vi "Weird Slave.vi"() -> ()   [LabVIEW 2012]
uses:
  API/Slave/Modbus Slave.lvclass
  Data Model/Standard Data Model/Standard Data Model.lvclass
  Transmission Data Unit/RTU/RTU Data Unit.lvclass
  Transmission Data Unit/ASCII/ASCII Data Unit.lvclass
  Network Protocol/Network Slave/TCP/TCP Slave.lvclass
  Transmission Data Unit/Serial Interface/Serial Data Unit.lvclass
  Data Model/Identification Parameters.ctl
  Data Model/Device Data Model.lvclass
  Master Function Definition/Read Device ID code.ctl
panel:
  in  "Port":u16=502
  in  "Serial Type":enum16{"RTU", "ASCII"}(ring)
  in  "Unit ID":u8=1
  in  "HR to write":u16[](array[numeric])=[1, 65535, 40000, 20000]
  in  "Set HR":bool
  in  "Set IR":bool
  in  "IR to write":u16[](array[numeric])=[1, 65535, 40000, 20000]
  in  "IR 6":u16
  in  "Set !":bool
  in  "! status":u8=1
  in  "Set Coils":bool
  in  "Set DI":bool
  in  "DI to write":bool[](array[boolean])=[FALSE, TRUE, FALSE, TRUE]
  in  "coils to write":bool[](array[boolean])=[FALSE, TRUE, FALSE, TRUE]
  in  "set objects":bool
  in  "Objects In":T1[](array[typedef])=[{"Object ID"=0, "Value"="National instruments"}, {"Object ID"=1, "Value"="42"}, {"Object ID"=2, "Value"="1.0.0"}] {"Object ID" format="%x"}
  in  "Coil 6":bool
  out "exception status":u8=1
  out "register values":u16[](array[numeric])=[1, 1, 65535, 40000, 20000, 6]
  out "discrete inputs":bool[](array[boolean])=[FALSE, FALSE, TRUE, FALSE, TRUE, TRUE]
  in  "Read Device ID code":T2
  out "Objects":T1[](array[typedef])=[{"Object ID"=0, "Value"="National instruments"}, {"Object ID"=1, "Value"="42"}, {"Object ID"=2, "Value"="1.0.0"}] {"Object ID" format="%x"}
  in  "Object Id":u8 format="%02x"
  out "holding reg":u16[](array[numeric])=[1, 1, 65535, 40000, 20000, 6]
  out "error out":errorcluster
  in  "stop":bool
  out "Coils":bool[](array[boolean])=[FALSE, FALSE, TRUE, FALSE, TRUE, TRUE] caption="Coils (Master can write coils)"
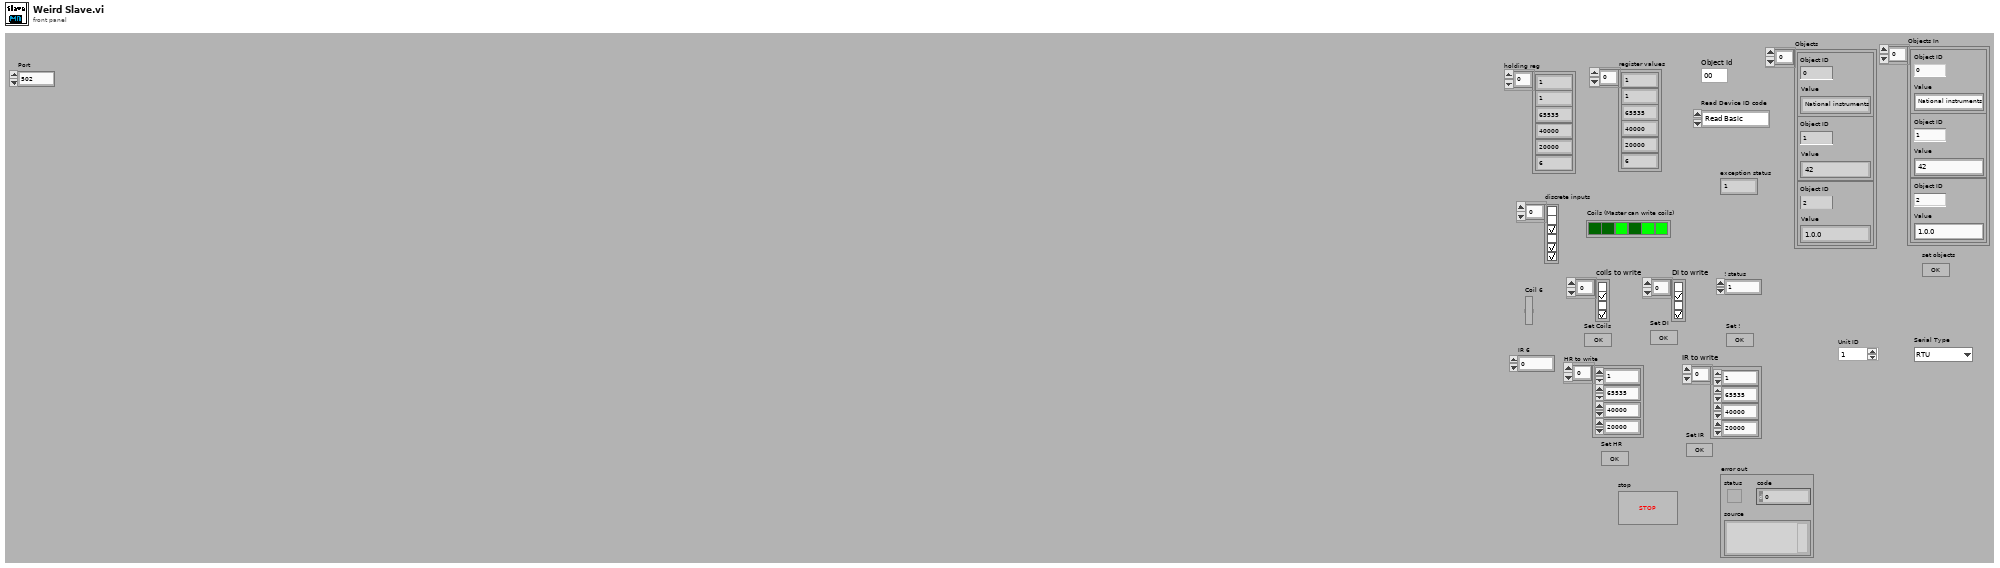
[diagram p1: front panel]
types:
  T1 = typedef "Device Data Model.lvclass/Identification Parameters.ctl" = cluster{"Object ID":u8, "Value":string}
  T2 = typedef "Device Data Model.lvclass/Read Device ID code.ctl" = enum8{"Read Basic", "Read Regular", "Read Extended", "Read Specific"}
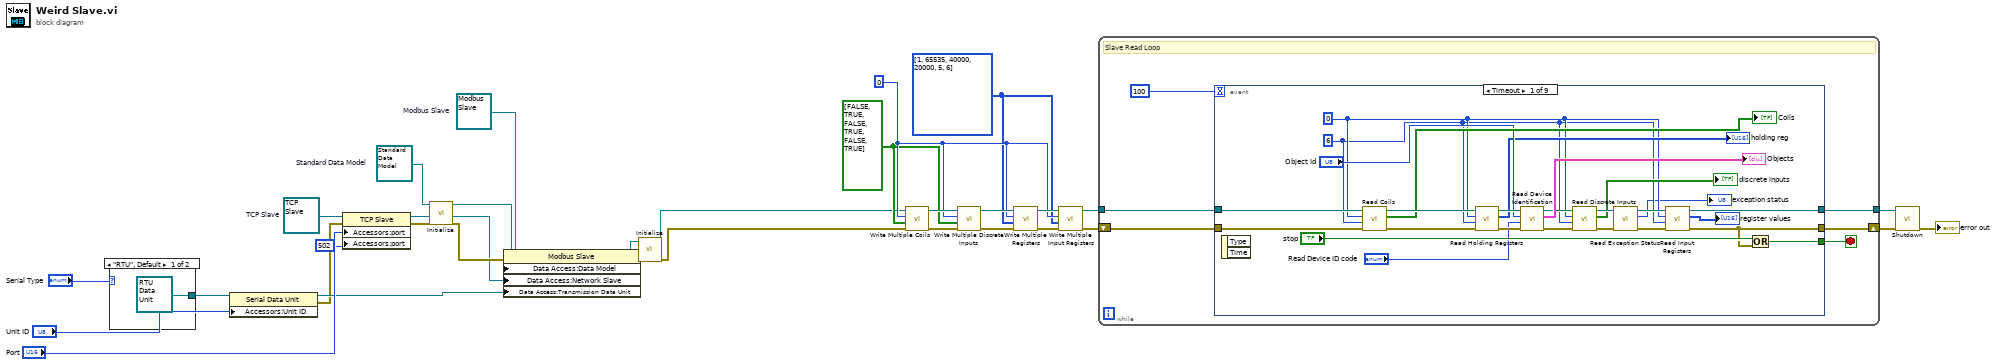
[diagram p0: block diagram]
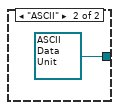
[diagram p2: hidden frame]
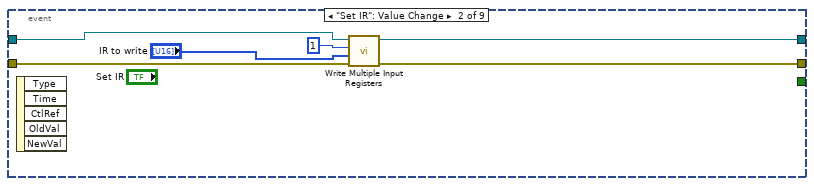
[diagram p3: hidden frame]
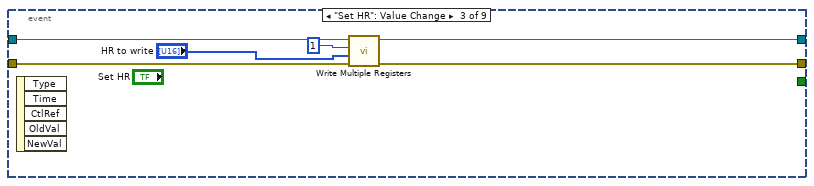
[diagram p4: hidden frame]
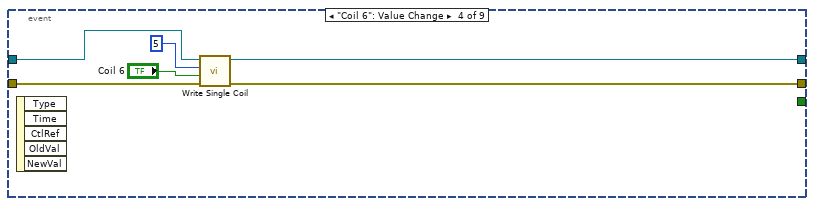
[diagram p5: hidden frame]
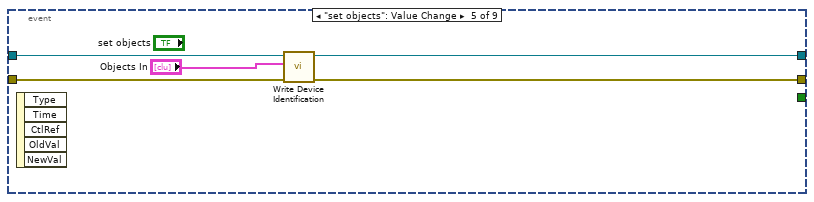
[diagram p6: hidden frame]
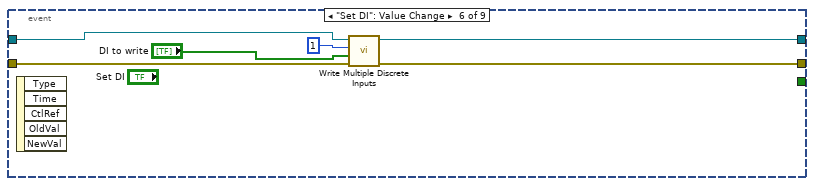
[diagram p7: hidden frame]
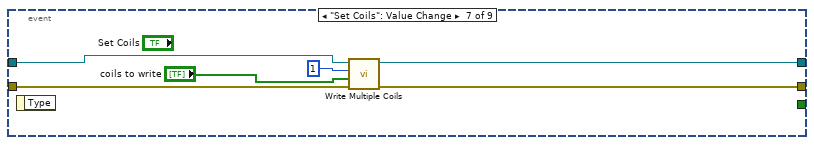
[diagram p8: hidden frame]
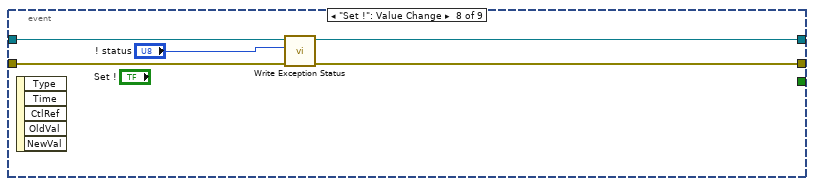
[diagram p9: hidden frame]
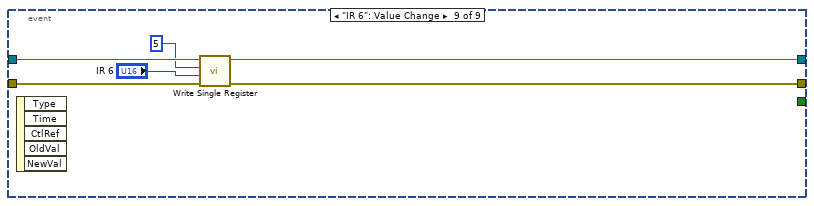
[diagram p10: hidden frame]
diagram:
  w4 = refnum<class "Standard Data Model.lvclass"> refnum  # Standard Data Model
  w15 = refnum<class "TCP Slave.lvclass"> refnum  # TCP Slave
  w13 = refnum<class "Modbus Slave.lvclass"> refnum  # Modbus Slave
  w19 = bool[] [FALSE, TRUE, FALSE, TRUE, FALSE, TRUE] ("coils to write")
  w20 = u16[] [1, 65535, 40000, 20000, 5, 6] ("registers")
  w21 = u16 0 ("starting address")
  n1 = case shown="\"RTU\", Default" "Serial Type" {
    tunnel: [refnum<class "RTU Data Unit.lvclass"> refnum ("RTU Data Unit") refnum<class "ASCII Data Unit.lvclass"> refnum ("ASCII Data Unit")] -> w17
    frame "RTU", Default {
    }
    frame "ASCII" {
    }
  }
  n2 = property class="Serial Data Unit"(reference=w17, "Accessors:Unit ID"="Unit ID") -> (reference out=w5:refnum<class "Serial Data Unit.lvclass">, error out=w3:errorcluster)  [unwired: 1 in]
  n3 = property class="TCP Slave"(reference=w15, error in=w3, "Accessors:port"="Port", "Accessors:port"=u16 502 ("Port")) -> (reference out=w11:refnum<class "TCP Slave.lvclass">, error out=w8:errorcluster)
  n4 = call-dynamic "Initialize.vi"("error in"=w8, "device data model in"=w4) -> ("error out"=w12:errorcluster, "device data model out"=w1:refnum<class "Standard Data Model.lvclass">)  [unwired: 8 in]
  n5 = property class="Modbus Slave"(reference=w13, error in=w12, "Data Access:Data Model"=w1, "Data Access:Network Slave"=w11, "Data Access:Transmission Data Unit"=w5) -> (reference out=w9:refnum<class "Modbus Slave.lvclass">, error out=w10:errorcluster)
  n6 = call-dynamic "Initialize.vi"("error in"=w10, "Modbus slave in"=w9) -> ("error out"=w6:errorcluster, "Modbus slave out"=w7:refnum<class "Modbus Slave.lvclass">)  [unwired: 8 in]
  n7 = call-dynamic "Write Multiple Coils.vi"("error in"=w6, "coils to write"=w19, "starting address"=w21, "Modbus slave in"=w7) -> ("error out"=w24:errorcluster, "Modbus slave out"=w25:refnum<class "Modbus Slave.lvclass">)  [unwired: 6 in]
  n8 = call-dynamic "Write Multiple Discrete Inputs.vi"("error in"=w24, "discrete inputs to write"=w19, "starting address"=w21, "Modbus slave in"=w25) -> ("error out"=w27:errorcluster, "Modbus slave out"=w26:refnum<class "Modbus Slave.lvclass">)  [unwired: 6 in]
  n9 = call-dynamic "Write Multiple Registers.vi"("error in"=w27, "registers to write"=w20, "starting address"=w21, "Modbus slave in"=w26) -> ("error out"=w28:errorcluster, "Modbus slave out"=w29:refnum<class "Modbus Slave.lvclass">)  [unwired: 6 in]
  n10 = call-dynamic "Write Multiple Input Registers.vi"("error in"=w28, "input registers to write"=w20, "starting address"=w21, "Modbus slave in"=w29) -> ("error out"=w23:errorcluster, "Modbus slave out"=w22:refnum<class "Modbus Slave.lvclass">)  [unwired: 6 in]
  n11 = while {
    tunnel: [w36] -> w32
    tunnel: w22 -> [w39]
    shift-right: [w37] -> w31
    shift-left: w23 -> [w38]
    stop <- w40 stop-if-true
    # "Slave Read Loop"
    n12 = event shown="[0] Timeout" {
      selector: _ -> [_ _ _ _ _ _ _ _ _]
      dyn-events: _ -> [_ _ _ _ _ _ _ _ _]
      timeout: 100 -> [_ _ _ _ _ _ _ _ _]
      tunnel: [w63 _ _ _ _ _ _ _ _] -> w40
      tunnel: w39 -> [w58 w69 w78 w81 w86 w95 w98 w105 w112]
      tunnel: w38 -> [w57 w70 w75 w82 w87 w94 w99 w106 w111]
      tunnel: [w53 w71 w76 w83 w88 w91 w100 w103 w110] -> w37
      tunnel: [w52 w72 w77 w84 w89 w90 w101 w102 w109] -> w36
      event Timeout {
        w43 = u16 6 ("Number of coils")
        w44 = u16 0 ("Starting Address")
        n13 = event-data() -> ()  [unwired: 1 in, 2 out]
        n14 = call-dynamic "Read Coils.vi"("error in"=w57, "number of inputs"=w43, "starting address"=w44, "Modbus slave in"=w58) -> ("error out"=w62:errorcluster, "coils"=→"Coils":bool[], "Modbus slave out"=w61:refnum<class "Modbus Slave.lvclass">)  [unwired: 5 in]
        n15 = call-dynamic "Read Holding Registers.vi"("error in"=w62, "number of inputs"=w43, "starting address"=w44, "Modbus slave in"=w61) -> ("error out"=w64:errorcluster, "register values"=→"holding reg":u16[], "Modbus slave out"=w65:refnum<class "Modbus Slave.lvclass">)  [unwired: 5 in]
        n16 = call-dynamic "Read Device Identification.vi"("error in"=w64, "read device ID code"="Read Device ID code", "object ID"="Object Id", "Modbus slave in"=w65) -> ("error out"=w49:errorcluster, "objects"=→"Objects":T1[], "Modbus slave out"=w46:refnum<class "Modbus Slave.lvclass">)  [unwired: 5 in]
        n17 = call-dynamic "Read Discrete Inputs.vi"("error in"=w49, "number of inputs"=w43, "starting address"=w44, "Modbus slave in"=w46) -> ("error out"=w50:errorcluster, "discrete inputs"=→"discrete inputs":bool[], "Modbus slave out"=w48:refnum<class "Modbus Slave.lvclass">)  [unwired: 5 in]
        n18 = call-dynamic "Read Exception Status.vi"("error in"=w50, "Modbus slave in"=w48) -> ("error out"=w51:errorcluster, "exception status"=→"exception status":u8, "Modbus slave out"=w47:refnum<class "Modbus Slave.lvclass">)  [unwired: 7 in]
        n19 = call-dynamic "Read Input Registers.vi"("error in"=w51, "number of inputs"=w43, "starting address"=w44, "Modbus slave in"=w47) -> ("error out"=w53:errorcluster, "register values"=→"register values":u16[], "Modbus slave out"=w52:refnum<class "Modbus Slave.lvclass">)  [unwired: 5 in]
        n20 = Or(x="stop", y=w53) -> (x .or. y?=w63:bool)
      }
      event "Set IR": Value Change {
        n21 = event-data() -> ()  [unwired: 1 in, 5 out]
        n22 = call-dynamic "Write Multiple Input Registers.vi"("error in"=w70, "input registers to write"="IR to write", "starting address"=u16 1, "Modbus slave in"=w69) -> ("error out"=w71:errorcluster, "Modbus slave out"=w72:refnum<class "Modbus Slave.lvclass">)  [unwired: 6 in]
      }
      event "Set HR": Value Change {
        n23 = event-data() -> ()  [unwired: 1 in, 5 out]
        n24 = call-dynamic "Write Multiple Registers.vi"("error in"=w75, "registers to write"="HR to write", "starting address"=u16 1, "Modbus slave in"=w78) -> ("error out"=w76:errorcluster, "Modbus slave out"=w77:refnum<class "Modbus Slave.lvclass">)  [unwired: 6 in]
      }
      event "Coil 6": Value Change {
        n25 = event-data() -> ()  [unwired: 1 in, 5 out]
        n26 = call-dynamic "Write Single Coil.vi"("error in"=w82, "coil to write"="Coil 6", "address"=u16 5, "Modbus slave in"=w81) -> ("error out"=w83:errorcluster, "Modbus slave out"=w84:refnum<class "Modbus Slave.lvclass">)  [unwired: 6 in]
      }
      event "set objects": Value Change {
        n27 = event-data() -> ()  [unwired: 1 in, 5 out]
        n28 = call-dynamic "Write Device Identification.vi"("error in"=w87, "objects"="Objects In", "Modbus slave in"=w86) -> ("error out"=w88:errorcluster, "Modbus slave out"=w89:refnum<class "Modbus Slave.lvclass">)  [unwired: 7 in]
      }
      event "Set DI": Value Change {
        n29 = event-data() -> ()  [unwired: 1 in, 5 out]
        n30 = call-dynamic "Write Multiple Discrete Inputs.vi"("error in"=w94, "discrete inputs to write"="DI to write", "starting address"=u16 1, "Modbus slave in"=w95) -> ("error out"=w91:errorcluster, "Modbus slave out"=w90:refnum<class "Modbus Slave.lvclass">)  [unwired: 6 in]
      }
      event "Set Coils": Value Change {
        n31 = event-data() -> ()  [unwired: 1 in, 1 out]
        n32 = call-dynamic "Write Multiple Coils.vi"("error in"=w99, "coils to write"="coils to write", "starting address"=u16 1, "Modbus slave in"=w98) -> ("error out"=w100:errorcluster, "Modbus slave out"=w101:refnum<class "Modbus Slave.lvclass">)  [unwired: 6 in]
      }
      event "Set !": Value Change {
        n33 = event-data() -> ()  [unwired: 1 in, 5 out]
        n34 = call "Write Exception Status.vi"("error in"=w106, "exception status"="! status", "Modbus slave in"=w105) -> ("error out"=w103:errorcluster, "Modbus slave out"=w102:refnum<class "Modbus Slave.lvclass">)  [unwired: 7 in]
      }
      event "IR 6": Value Change {
        n35 = event-data() -> ()  [unwired: 1 in, 5 out]
        n36 = call-dynamic "Write Single Register.vi"("error in"=w111, "register to write"="IR 6", "address"=u16 5, "Modbus slave in"=w112) -> ("error out"=w110:errorcluster, "Modbus slave out"=w109:refnum<class "Modbus Slave.lvclass">)  [unwired: 6 in]
      }
    }
  }
  n37 = call-dynamic "Shutdown.vi"("error in"=w31, "Modbus slave in"=w32) -> ("error out"=→"error out":errorcluster)  [unwired: 9 in]
